vi "Calculate Entropy.vi"(8 "error in (no error)":errorcluster, 11 "GA in":refnum<class "GA.lvclass">) -> (0 "error out":errorcluster, 2 "Unique Fitness Values":i32, 3 "Entropy Out":dbl)   [LabVIEW 2013]
uses:
  Classes/GA.lvclass
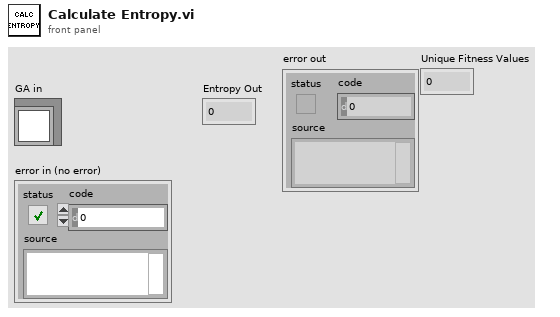
[diagram p1: front panel]
types:
  T1 = typedef "Solution_GA.ctl" = cluster{"Schedule":u16[], "Fitness":u16, "Fitness Valid?":bool}
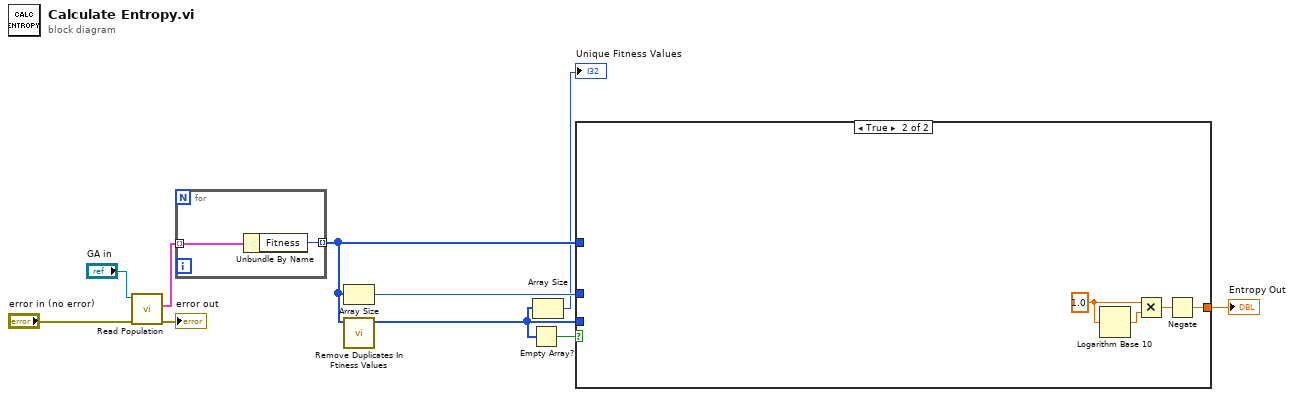
[diagram p0: block diagram]
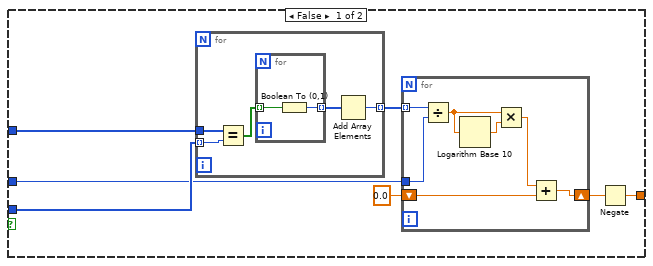
[diagram p2: hidden frame]
diagram:
  n1 = call-dynamic "Read Population.vi"("error in (no error)"="error in (no error)", "GA in"="GA in") -> ("error out"=→"error out":errorcluster, "Population"=w8:T1[])  [unwired: 7 in, 1 out]
  n2 = for {
    tunnel: w8 -> [w12] mode=indexing
    tunnel: [w11] -> w7 mode=indexing
    n3 = Unbundle By Name(w12) -> ("Fitness"=w11:u16)
  }
  n4 = Array Size(array=w7) -> (size(s)=w6:i32)
  n5 = call "Remove Duplicates In Ftiness Values.vi"("Fitness Values In"=w7) -> ("Unique Fitness Values Out"=w2:u16[])  [unwired: 10 in]
  n6 = Empty Array?(array=w2) -> (empty?=w3:bool)
  n7 = Array Size(array=w2) -> (size(s)=→"Unique Fitness Values":i32)
  n8 = case shown="True" w3 {
    tunnel: w2 -> [w19 _]
    tunnel: w7 -> [w18 _]
    tunnel: w6 -> [w17 _]
    tunnel: [w13 w34] -> w4
    frame False {
      n9 = for {
        tunnel: w19 -> [w30] mode=indexing
        tunnel: w18 -> [w31]
        tunnel: [w27] -> w16 mode=indexing
        n10 = Equal?(x=w31, y=w30) -> (x = y?=w29:bool[])
        n11 = for {
          tunnel: w29 -> [w33] mode=indexing
          tunnel: [w32] -> w28 mode=indexing
          n12 = Boolean To (0,1)(Boolean=w33) -> (0, 1=w32:i16)
        }
        n13 = Add Array Elements(numeric array=w28) -> (sum=w27:i16)
      }
      n14 = for {
        tunnel: w17 -> [w25]
        tunnel: w16 -> [w26] mode=indexing
        shift-right: [w20] -> w14
        shift-left: 0.0 -> [w21]
        n15 = Divide(x=w26, y=w25) -> (x/y=w24:dbl)
        n16 = Logarithm Base 10(1:w24) -> (0:w23:dbl)
        n17 = Multiply(x=w24, y=w23) -> (x*y=w22:dbl)
        n18 = Add(x=w22, y=w21) -> (x+y=w20:dbl)
      }
      n19 = Negate(x=w14) -> (-x=w13:dbl)
    }
    frame True {
      w37 = 1.0
      n20 = Logarithm Base 10(1:w37) -> (0:w36:dbl)
      n21 = Multiply(x=w37, y=w36) -> (x*y=w35:dbl)
      n22 = Negate(x=w35) -> (-x=w34:dbl)
    }
  }
  "Entropy Out" <- w4
